vi "niFPGA Switch_m.vi"   [LabVIEW 2017]
doc: "Switches between two input values based on the value of <B>control input</B>. The data type you wire to <B>input 1</B> or <B>input 2</B> determines the <B>output</B> data type."
uses:
  <vilib>/rvi/Analysis/common/FxpNativeNode/niFpgaFxpNative.xnode
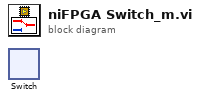
[diagram p0: block diagram]
diagram:
  n1 = xnode ("Switch")() -> ()  [unwired: 4 in, 1 out]
